vi "height_map_to_3D_scene_TOF_.vi"(5 "min value":dbl=40.0 format="%#_13g", 6 "Reflectivity":dbl[][](array[numeric]), 7 "max value":dbl=80.0 format="%#_13g", 8 "Height Map":dbl[][](array[numeric])) -> (0 "Height":T1, 1 "Reflectivity":T1, 2 "3D Scene (textured)":refnum<vi>, 3 "3D Scene (height map)":refnum<vi>)   [LabVIEW 2020]
uses:
  <vilib>/picture/picture.llb/imagedata.ctl
  <vilib>/picture/3D Picture Control/Object/Create Object (name).vi
  <vilib>/picture/3D Picture Control/NI_3D Picture Control.lvlib
panel:
  in  "image data":T1
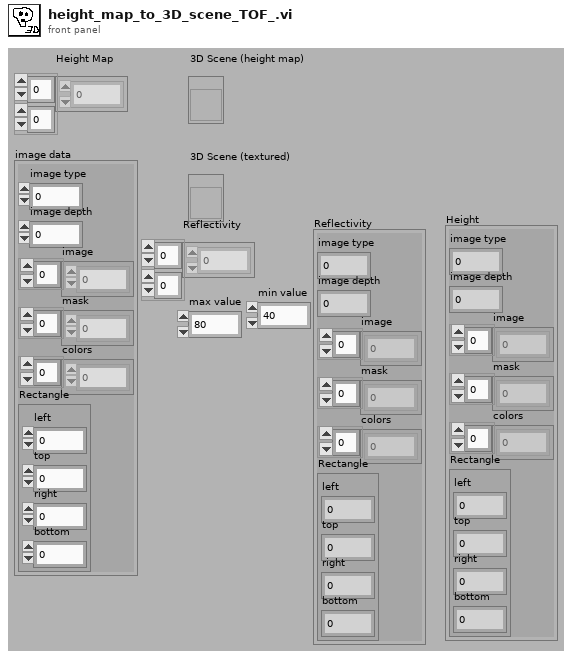
[diagram p1: front panel]
types:
  T1 = typedef "imagedata.ctl" = cluster{"image type":i32, "image depth":i32, "image":u8[], "mask":u8[], "colors":u32[], "Rectangle":cluster{"left":i16, "top":i16, "right":i16, "bottom":i16}}
  T2 = enum16{"Gray", "RGB", "CMY", "Black -> Blue -> White", "Custom", "HSL"}
  T3 = enum16{"Inherit Value", "Points", "Wireframe", "Polygons"}
  T4 = cluster{"Red":sgl, "Green":sgl, "Blue":sgl, "Alpha":sgl}
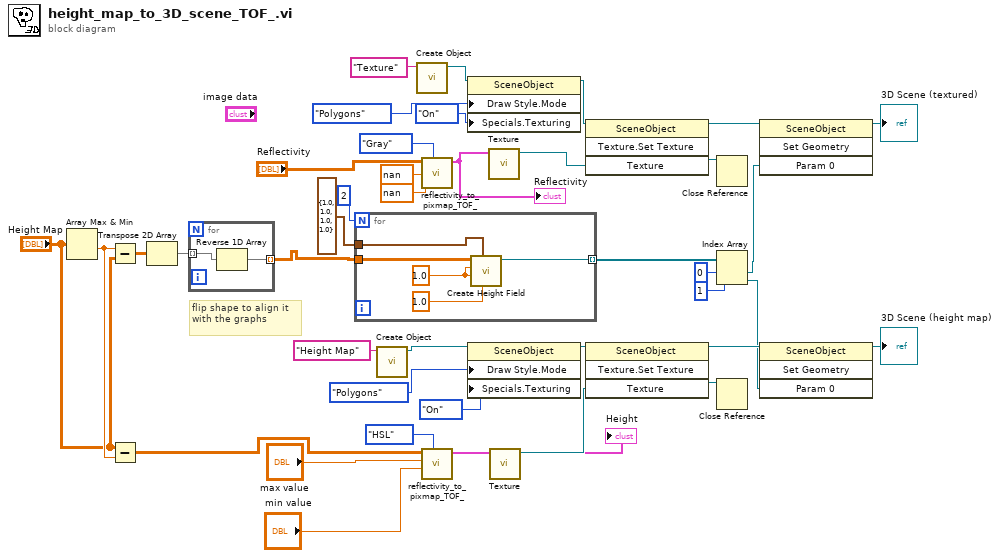
[diagram p0: block diagram]
diagram:
  # "flip shape to align it with the graphs"
  n1 = Array Max & Min(array="Height Map") -> (min value=w17:dbl)  [unwired: 3 out]
  n2 = Subtract(x=w17, y="Height Map") -> (x-y=w2:dbl[][])
  n3 = Subtract(x="Height Map", y=w17) -> (x-y=w4:dbl[][])
  n4 = Transpose 2D Array(2D array=w2) -> (transposed array=w37:dbl[][])
  n5 = for {
    tunnel: w37 -> [w42] mode=indexing
    tunnel: [w41] -> w1 mode=indexing
    n6 = Reverse 1D Array(array=w42) -> (reversed array=w41:dbl[])
  }
  n7 = for {
    N: 2 -> [_]
    tunnel: [w47] -> w33 mode=indexing
    tunnel: T4 {"Red"=1.0, "Green"=1.0, "Blue"=1.0, "Alpha"=1.0} ("Color") -> [w46]
    tunnel: w1 -> [w45]
    w44 = sgl 1.0 ("Row Interval")
    n8 = call <vilib>:"Create Height Field.vi"("Base Height"=sgl 1.0, "Color"=w46, "Column Interval"=w44, "Row Interval"=w44, "Data"=w45) -> ("New Height Field Refnum"=w47:refnum<vi>)  [unwired: 5 in, 1 out]
  }
  n9 = call-poly <vilib>:"Create Object.vi"("Name"="Height Map") -> ("Scene:New Object"=w32:refnum<vi>)  [unwired: 9 in, 1 out]
  n10 = call-poly <vilib>:"Create Object.vi"("Name"="Texture") -> ("Scene:New Object"=w23:refnum<vi>)  [unwired: 9 in, 1 out]
  n11 = call "reflectivity_to_pixmap_TOF_.vi"("colours"=T2."Gray", "min value"=nan, "max value"=nan, "DBL Array"="Reflectivity") -> ("image data"=w11:T1)  [unwired: 6 in]
  "Reflectivity" <- w11
  n12 = call "reflectivity_to_pixmap_TOF_.vi"("colours"=T2."HSL", "min value"="min value", "max value"="max value", "DBL Array"=w4) -> ("image data"=w22:T1)  [unwired: 6 in]
  "Height" <- w22
  n13 = property class="SceneObject"(reference=w23, "Draw Style.Mode"=T3."Polygons" ("Draw Style:Mode"), "Specials.Texturing"=enum16{"Inherit Value", "Off", "On"}."On" ("Specials:Texturing")) -> (reference out=w26:refnum<vi>)  [unwired: 1 in, 1 out]
  n14 = property class="SceneObject"(reference=w32, "Draw Style.Mode"=T3."Polygons" ("Draw Style:Mode"), "Specials.Texturing"=enum16{"Inherit Value", "Off", "On"}."On" ("Specials:Texturing")) -> (reference out=w29:refnum<vi>)  [unwired: 1 in, 1 out]
  n15 = call <vilib>:"Texture.vi"("Image"=w11) -> ("New Texture Refnum"=w35:refnum<vi>)  [unwired: 1 in, 9 out]
  n16 = call <vilib>:"Texture.vi"("Image"=w22) -> ("New Texture Refnum"=w34:refnum<vi>)  [unwired: 1 in, 9 out]
  n17 = invoke class="SceneObject" method="Texture.Set Texture"(reference=w26, "Texture"=w35) -> (reference out=w25:refnum<vi>, "Texture"=w21:refnum<vi>)  [unwired: 2 in, 2 out]
  n18 = invoke class="SceneObject" method="Texture.Set Texture"(reference=w29, "Texture"=w34) -> (reference out=w30:refnum<vi>, "Texture"=w20:refnum<vi>)  [unwired: 2 in, 2 out]
  n19 = Close Reference(reference=w21) -> ()  [unwired: 1 in, 1 out]
  n20 = Index Array(array=w33, index #1=0 ("index"), index #2=1 ("index")) -> (element #1=w14:refnum<vi>, element #2=w13:refnum<vi>)
  n21 = Close Reference(reference=w20) -> ()  [unwired: 1 in, 1 out]
  n22 = invoke class="SceneObject" method="Set Geometry"(reference=w25, "Param 0"=w14) -> (reference out=→"3D Scene (textured)":refnum<vi>)  [unwired: 2 in, 3 out]
  n23 = invoke class="SceneObject" method="Set Geometry"(reference=w30, "Param 0"=w13) -> (reference out=→"3D Scene (height map)":refnum<vi>)  [unwired: 2 in, 3 out]
